vi "RunAppleScriptCode.vi"(8 "Error In":errorcluster, 9 "Run Later":bool=TRUE, 10 "wait until completion? (T)":bool=TRUE, 11 "Input String":string="tell application \"Finder\"\nactivate\ndisplay dialog \"LabVIEW is talking to you\"\nend tell\n") -> (0 "Error Out":errorcluster, 2 "Compile & Runtime Errors":string, 3 "Results":string)   [LabVIEW 2010]
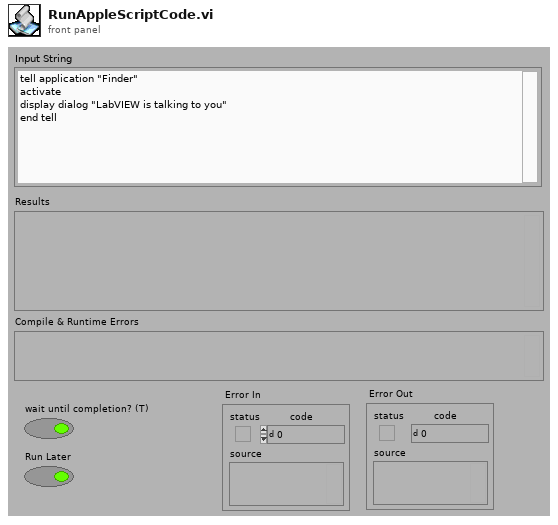
[diagram p1: front panel]
types:
  T1 = enum16{"Native", "Native Command Line", "UNIX", "Macintosh", "DOS"}
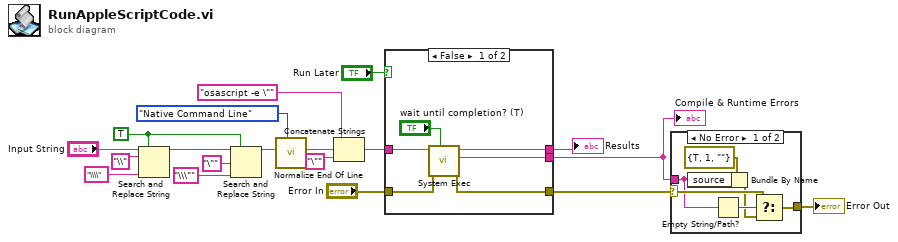
[diagram p0: block diagram]
diagram:
  w4 = TRUE ("replace all? (F)")
  n1 = Search and Replace String(replace all?=w4, input string="Input String", search string="\\", replace string="\\\\" ("replace string (\"\")")) -> (result string=w5:string)  [unwired: 4 in, 3 out]
  n2 = Search and Replace String(replace all?=w4, input string=w5, search string="\"", replace string="\\\"" ("replace string (\"\")")) -> (result string=w17:string)  [unwired: 4 in, 3 out]
  n3 = call <vilib>:"Normalize End Of Line.vi"("End Of Line (Native)"=T1."Native Command Line", "String In"=w17) -> ("String Out"=w15:string)  [unwired: 6 in]
  n4 = Concatenate Strings("osascript -e \"" ("string"), w15, "\"" ("string")) -> (w12:string)
  n5 = case shown="False" "Run Later" {
    tunnel: w12 -> [w25 w27]
    tunnel: "Error In" -> [w24 w26]
    tunnel: [w23 w27] -> w10
    tunnel: [w22 w26] -> w9
    tunnel: [w21 _] -> w8
    frame False {
      n6 = call <vilib>:"System Exec.vi"("wait until completion? (T)"="wait until completion? (T)", "error in (no error)"=w24, "command line"=w25) -> ("error out"=w22:errorcluster, "standard error"=w21:string, "standard output"=w23:string)  [unwired: 5 in, 1 out]
    }
    frame True {
    }
  }
  "Results" <- w10
  "Compile & Runtime Errors" <- w8
  n7 = case shown="No Error" w9 {
    selector: w9 -> [w31 w34]
    tunnel: w8 -> [w30 _]
    tunnel: [w28 w34] -> w7
    frame No Error {
      n8 = Bundle By Name(cluster=errorcluster {"status"=TRUE, "code"=1, "source"=""} ("error IO"), "source"=w30) -> (w29:errorcluster)
      n9 = Empty String/Path?(string/path=w30) -> (empty?=w32:bool)
      n10 = Select(t=w31, s=w32, f=w29) -> (s? t:f=w28:errorcluster)
    }
    frame Error {
    }
  }
  "Error Out" <- w7
